vi "Power Spectrum.vi"(0 "X":dbl[](array[numeric]) format="%.2f") -> (1 "Power Spectrum":dbl[](array[numeric]) format="%.2f", 2 "error":i32)   [LabVIEW 2009]
doc: "Computes the <B>Power Spectrum</B>, Sxx, of the input sequence <B>X</B>."
uses:
  C:/Program Files/National Instruments/LabVIEW 2009/resource/lvanlys.dll
panel:
  # "Power Spectrum"
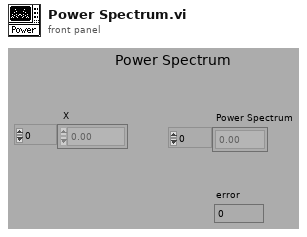
[diagram p1: front panel]
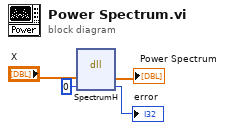
[diagram p0: block diagram]
diagram:
  n1 = dll-call lib="C:/Program Files/National Instruments/LabVIEW 2009/resource/lvanlys.dll" fn="SpectrumH"("X"="X", "error"=0) -> ("X"=→"Power Spectrum":dbl[], "error"=→"error":i32)  [unwired: 4 in, 2 out]
